vi "Get I32.vi"(8 "error in (no error)":errorcluster, 11 "I32Msg in":refnum<class "I32Msg.lvclass">) -> (0 "error out":errorcluster, 2 "Message Data":i32, 3 "I32Msg out":refnum<class "I32Msg.lvclass">)   [LabVIEW 2017, in "LapDog.Messaging.v3.NativeTypes.lvlib" / "I32Msg.lvclass"]
doc: "Returns the data contained in the message.\n\nThis method executes regardless of the error in state."
uses:
  I32Msg.lvclass
  I32Msg.lvclass/I32Msg.ctl
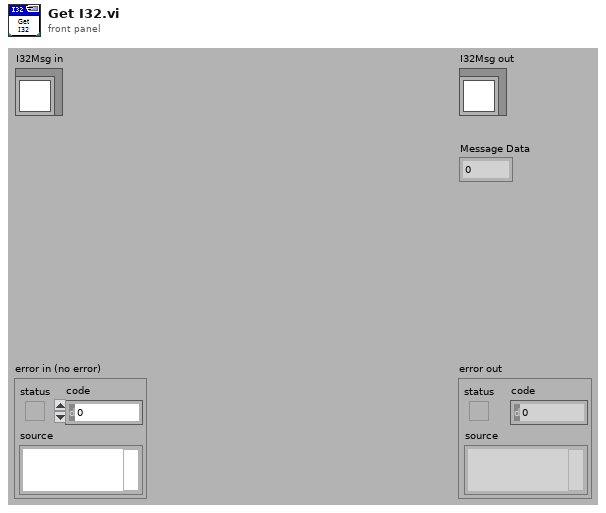
[diagram p1: front panel]
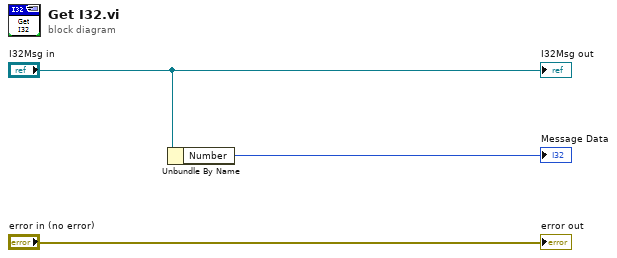
[diagram p0: block diagram]
diagram:
  n1 = Unbundle By Name("I32Msg in") -> ("Number"=→"Message Data":i32)
  "error out" <- "error in (no error)"
  "I32Msg out" <- "I32Msg in"
